vi "PathPlanner_Path_FlipPath.vi"(11 "in PathPlannerPath":T1={"Reversed"=FALSE, "RotationTargets"=[], "ConstraintZones"=[], "EventMarkers"=[], "GlobalConstraints"={"MaxVelocityMps;"=0.0, "MaxAccelerationMpsSq;"=0.0, "MaxAngularVelRadPsEc;"=0.0, "MaxAngularAccRadPSecSq"=0.0, "Exists"=FALSE, "Unlimited"=FALSE, "NominalVoltageVolts"=12.0}, "GoalEndState"={"VelocityMPS"=0.0, "Rotation"={"VALUE"=0.0, "COS"=1.0, "SIN"=0.0}}, "AllPoints"=[], "Name"="", "Waypoints"=[], "PointTowardsZones"=[], "IdealStartingState"={"VelocityMPS"=0.0, "Rotation"={"VALUE"=1.0, "COS"=0.0, "SIN"=0.0}, "NotNull"=FALSE}, "IsChoreoPath"=FALSE, "PreventFlipping"=FALSE} {"IdealStartingState"."Rotation"."SIN" format="%13.4f"; "IdealStartingState"."Rotation"."COS" format="%13.4f"; "IdealStartingState"."Rotation"."VALUE" format="%13.4f"; "PointTowardsZones"."TargetPosition"."Y" format="%14.3f"; "PointTowardsZones"."TargetPosition"."X" format="%14.3f"; "PointTowardsZones"."RotationOffset"."SIN" format="%13.4f"; "PointTowardsZones"."RotationOffset"."COS" format="%13.4f"; "PointTowardsZones"."RotationOffset"."VALUE" format="%13.4f"; "Waypoints"."nextControl"."Y" format="%14.3f"; "Waypoints"."nextControl"."X" format="%14.3f"; "Waypoints"."anchor"."Y" format="%14.3f"; "Waypoints"."anchor"."X" format="%14.3f"; "Waypoints"."prevControl"."Y" format="%14.3f"; "Waypoints"."prevControl"."X" format="%14.3f"; "AllPoints"."RotationTarget"."rotation"."SIN" format="%13.4f"; "AllPoints"."RotationTarget"."rotation"."COS" format="%13.4f"; "AllPoints"."RotationTarget"."rotation"."VALUE" format="%13.4f"; "AllPoints"."Position"."Y" format="%14.3f"; "AllPoints"."Position"."X" format="%14.3f"; "GoalEndState"."Rotation"."SIN" format="%13.4f"; "GoalEndState"."Rotation"."COS" format="%13.4f"; "GoalEndState"."Rotation"."VALUE" format="%13.4f"; "RotationTargets"."rotation"."SIN" format="%13.4f"; "RotationTargets"."rotation"."COS" format="%13.4f"; "RotationTargets"."rotation"."VALUE" format="%13.4f"}) -> (3 "out PathPlannerPath":T1={"Reversed"=FALSE, "RotationTargets"=[], "ConstraintZones"=[], "EventMarkers"=[], "GlobalConstraints"={"MaxVelocityMps;"=0.0, "MaxAccelerationMpsSq;"=0.0, "MaxAngularVelRadPsEc;"=0.0, "MaxAngularAccRadPSecSq"=0.0, "Exists"=FALSE, "Unlimited"=FALSE, "NominalVoltageVolts"=12.0}, "GoalEndState"={"VelocityMPS"=0.0, "Rotation"={"VALUE"=0.0, "COS"=1.0, "SIN"=0.0}}, "AllPoints"=[], "Name"="", "Waypoints"=[], "PointTowardsZones"=[], "IdealStartingState"={"VelocityMPS"=0.0, "Rotation"={"VALUE"=1.0, "COS"=0.0, "SIN"=0.0}, "NotNull"=FALSE}, "IsChoreoPath"=FALSE, "PreventFlipping"=FALSE} {"IdealStartingState"."Rotation"."SIN" format="%13.4f"; "IdealStartingState"."Rotation"."COS" format="%13.4f"; "IdealStartingState"."Rotation"."VALUE" format="%13.4f"; "PointTowardsZones"."TargetPosition"."Y" format="%14.3f"; "PointTowardsZones"."TargetPosition"."X" format="%14.3f"; "PointTowardsZones"."RotationOffset"."SIN" format="%13.4f"; "PointTowardsZones"."RotationOffset"."COS" format="%13.4f"; "PointTowardsZones"."RotationOffset"."VALUE" format="%13.4f"; "Waypoints"."nextControl"."Y" format="%14.3f"; "Waypoints"."nextControl"."X" format="%14.3f"; "Waypoints"."anchor"."Y" format="%14.3f"; "Waypoints"."anchor"."X" format="%14.3f"; "Waypoints"."prevControl"."Y" format="%14.3f"; "Waypoints"."prevControl"."X" format="%14.3f"; "AllPoints"."RotationTarget"."rotation"."SIN" format="%13.4f"; "AllPoints"."RotationTarget"."rotation"."COS" format="%13.4f"; "AllPoints"."RotationTarget"."rotation"."VALUE" format="%13.4f"; "AllPoints"."Position"."Y" format="%14.3f"; "AllPoints"."Position"."X" format="%14.3f"; "GoalEndState"."Rotation"."SIN" format="%13.4f"; "GoalEndState"."Rotation"."COS" format="%13.4f"; "GoalEndState"."Rotation"."VALUE" format="%13.4f"; "RotationTargets"."rotation"."SIN" format="%13.4f"; "RotationTargets"."rotation"."COS" format="%13.4f"; "RotationTargets"."rotation"."VALUE" format="%13.4f"})   [LabVIEW 2019, in "PathPlanner24.lvlib"]
doc: "Flip a path to the other side of the field, maintaining a global blue alliance origin\n\nInputs: \n - Path - cluster - path definition data structure\n\nOutputs:\n - Path - cluster - flipped path"
uses:
  PathPlanner24.lvlib
  TypeDef/PathPlannerPath.ctl
  TypeDef/PathPlannerRotationTarget.ctl
  <vilib>/Rock Robotics/WPI/ThirdParty/JAS_Junk/TrajLib/TypeDef/ROTATION2D.ctl
  TypeDef/PathPlannerConstraintsZone.ctl
  TypeDef/PathPlannerPathConstraints.ctl
  TypeDef/PathPlannerEventMarker.ctl
  TypeDef/PathPlannerCommandUtil.ctl
  ENum/PathPlanner_CommandUtil_Type_ENUM.ctl
  TypeDef/PathPlannerGoalEndState.ctl
  TypeDef/PathPlannerPathPoint.ctl
  <vilib>/Rock Robotics/WPI/ThirdParty/JAS_Junk/TrajLib/TypeDef/TRANSLATION2D.ctl
  TypeDef/PathPlannerWaypoint.ctl
  TypeDef/PathPlannerPointTowardsZone.ctl
  TypeDef/PathPlannerIdealStartingState.ctl
  PathPlanner_FieldUtil_FlipFieldPosition.vi
  PathPlanner_RotationTarget_New.vi
  PathPlanner_RotationTarget_GetAll.vi
  PathPlanner_FieldUtil_FlipFieldRotation.vi
  PathPlanner_FieldUtil_SymmetryType.vi
  PathPlanner_FieldUtil_FieldSizeY.vi
  <vilib>/Rock Robotics/WPI/ThirdParty/JAS_Junk/TrajLib/Translation2d_GetXY.vi
  <vilib>/Rock Robotics/WPI/ThirdParty/JAS_Junk/TrajLib/Translation2d_Create.vi
  PathPlanner_FieldUtil_FieldSizeX.vi
  <vilib>/Rock Robotics/WPI/ThirdParty/JAS_Junk/TrajLib/Rotation2d_CreateAngle.vi
  <vilib>/Rock Robotics/WPI/ThirdParty/JAS_Junk/TrajLib/Rotation2d_Minus.vi
  <vilib>/Rock Robotics/WPI/ThirdParty/JAS_Junk/TrajLib/Conv_Feet_Meters.vi
  <vilib>/Rock Robotics/WPI/ThirdParty/JAS_Junk/TrajLib/Rotation2d_UnaryMinus.vi
  <vilib>/Rock Robotics/WPI/ThirdParty/JAS_Junk/TrajLib/Rotation2d_RotateBy.vi
  <vilib>/Rock Robotics/WPI/ThirdParty/JAS_Junk/TrajLib/Rotation2d_CreateXY.vi
  <vilib>/Rock Robotics/WPI/ThirdParty/JAS_Junk/TrajLib/Util_CalcDist.vi
  <vilib>/Rock Robotics/WPI/ThirdParty/JAS_Junk/TrajLib/Trajectory_Library.lvlib
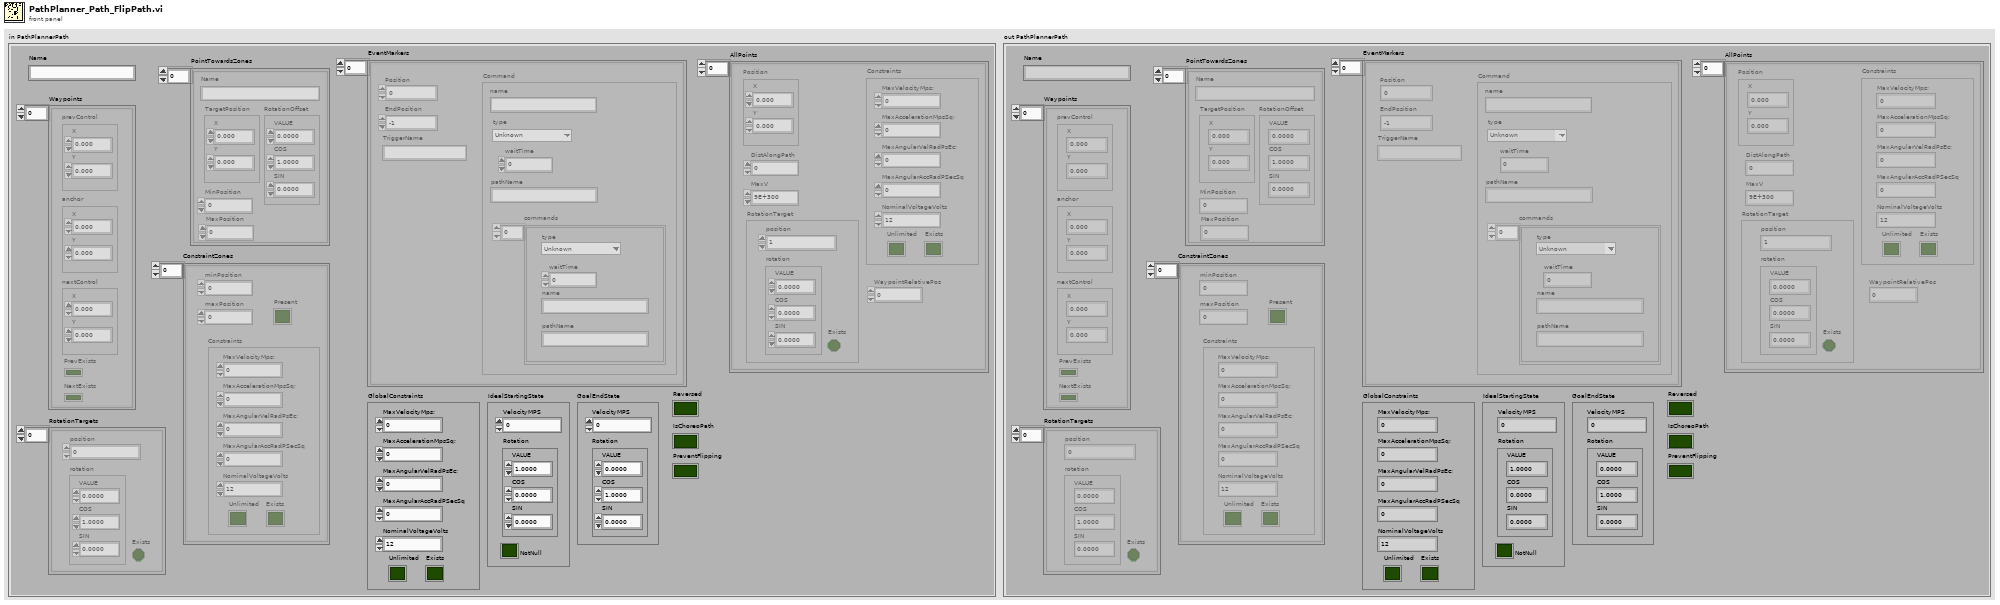
[diagram p1: front panel]
types:
  T1 = typedef "PathPlanner24.lvlib/PathPlannerPath.ctl" = cluster{"Reversed":bool, "RotationTargets":T2[], "ConstraintZones":T4[], "EventMarkers":T6[], "GlobalConstraints":T5, "GoalEndState":T9, "AllPoints":T10[], "Name":string, "Waypoints":T12[], "PointTowardsZones":T13[], "IdealStartingState":T14, "IsChoreoPath":bool, "PreventFlipping":bool}
  T2 = typedef "PathPlanner24.lvlib/PathPlannerRotationTarget.ctl" = cluster{"position":dbl, "rotation":T3, "Exists":bool}
  T3 = typedef "Trajectory_Library.lvlib/ROTATION2D.ctl" = cluster{"VALUE":dbl, "COS":dbl, "SIN":dbl}
  T4 = typedef "PathPlanner24.lvlib/PathPlannerConstraintsZone.ctl" = cluster{"minPosition":dbl, "maxPosition":dbl, "Constraints":T5, "Present":bool}
  T5 = typedef "PathPlanner24.lvlib/PathPlannerPathConstraints.ctl" = cluster{"MaxVelocityMps;":dbl, "MaxAccelerationMpsSq;":dbl, "MaxAngularVelRadPsEc;":dbl, "MaxAngularAccRadPSecSq":dbl, "Exists":bool, "Unlimited":bool, "NominalVoltageVolts":dbl}
  T6 = typedef "PathPlanner24.lvlib/PathPlannerEventMarker.ctl" = cluster{"Position":dbl, "Command":T7, "TriggerName":string, "EndPosition":dbl}
  T7 = typedef "PathPlanner24.lvlib/PathPlannerCommandUtil.ctl" = cluster{"waitTime":dbl, "name":string, "pathName":string, "commands":cluster{"type":T8, "waitTime":dbl, "name":string, "pathName":string}[], "type":T8}
  T8 = typedef "PathPlanner24.lvlib/PathPlanner_CommandUtil_Type_ENUM.ctl" = enum16{"Unknown", "Wait", "Named", "Path", "Sequential", "Parallel", "Race", "Deadline", "PointTowardsZoneEnter", "PointTowardsZoneExit", "TriggerEventStart", "TriggerEventStop", "TriggerEventOneshot"}
  T9 = typedef "PathPlanner24.lvlib/PathPlannerGoalEndState.ctl" = cluster{"VelocityMPS":dbl, "Rotation":T3}
  T10 = typedef "PathPlanner24.lvlib/PathPlannerPathPoint.ctl" = cluster{"Position":T11, "DistAlongPath":dbl, "MaxV":dbl, "Constraints":T5, "RotationTarget":T2, "WaypointRelativePos":dbl}
  T11 = typedef "Trajectory_Library.lvlib/TRANSLATION2D.ctl" = cluster{"X":dbl, "Y":dbl}
  T12 = typedef "PathPlanner24.lvlib/PathPlannerWaypoint.ctl" = cluster{"prevControl":T11, "anchor":T11, "nextControl":T11, "PrevExists":bool, "NextExists":bool}
  T13 = typedef "PathPlanner24.lvlib/PathPlannerPointTowardsZone.ctl" = cluster{"RotationOffset":T3, "Name":string, "TargetPosition":T11, "MinPosition":dbl, "MaxPosition":dbl}
  T14 = typedef "PathPlanner24.lvlib/PathPlannerIdealStartingState.ctl" = cluster{"VelocityMPS":dbl, "Rotation":T3, "NotNull":bool}
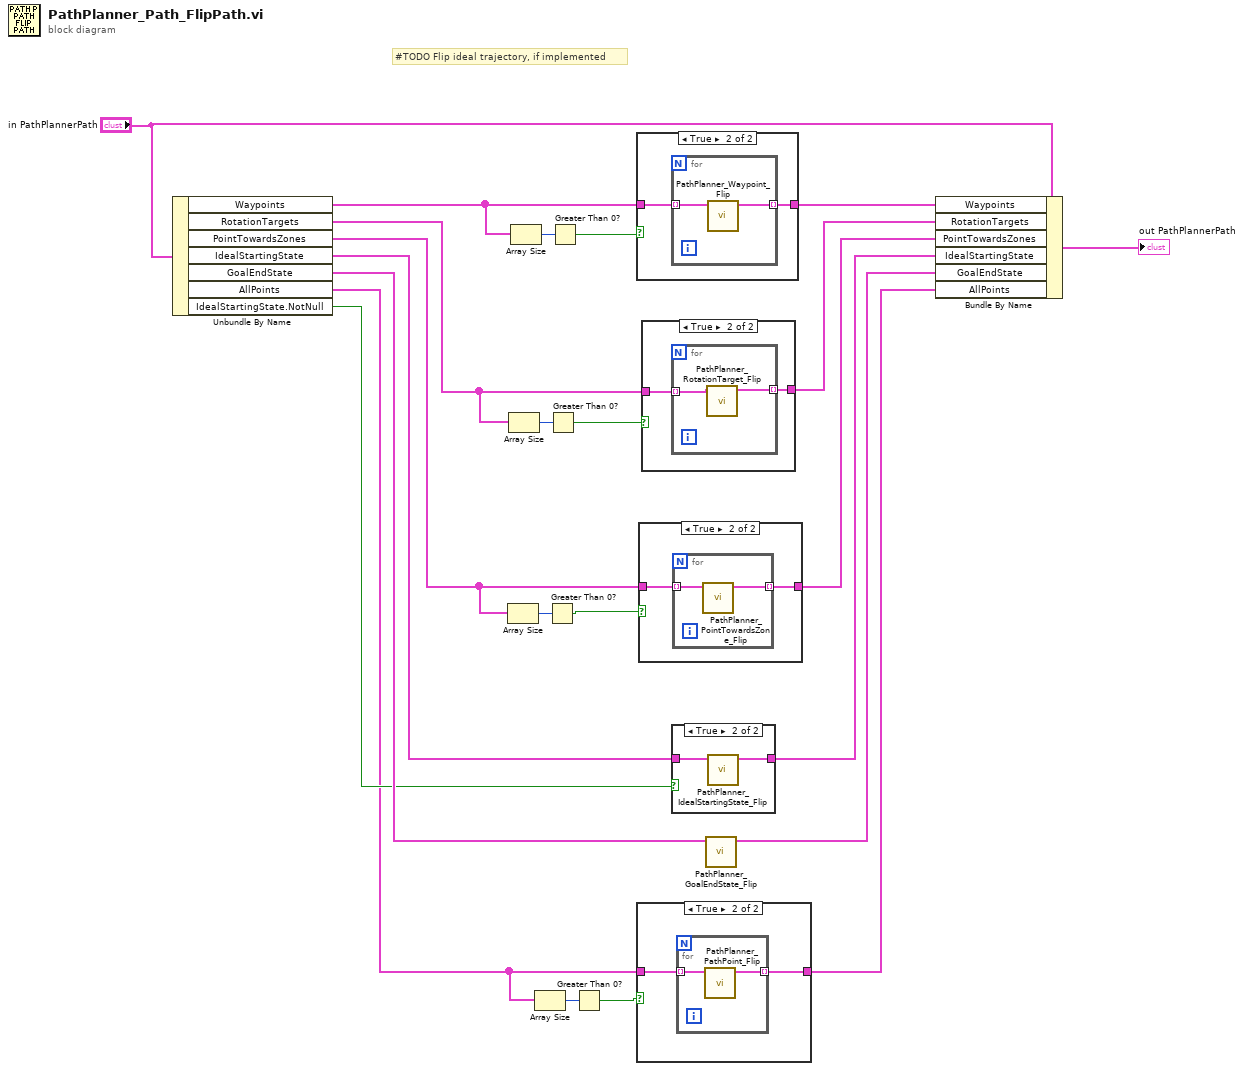
[diagram p0: block diagram]
diagram:
  # "#TODO Flip ideal trajectory, if implemented"
  n1 = Unbundle By Name("in PathPlannerPath") -> ("Waypoints"=w12:T12[], "RotationTargets"=w1:T2[], "PointTowardsZones"=w4:T13[], "IdealStartingState"=w18:T14, "GoalEndState"=w16:T9, "AllPoints"=w6:T10[], "IdealStartingState.NotNull"=w13:bool)
  n2 = Array Size(array=w4) -> (size(s)=w9:i32)
  n3 = Array Size(array=w1) -> (size(s)=w10:i32)
  n4 = Array Size(array=w12) -> (size(s)=w11:i32)
  n5 = Array Size(array=w6) -> (size(s)=w8:i32)
  n6 = Greater Than 0?(x=w9) -> (x > 0?=w5:bool)
  n7 = Greater Than 0?(x=w10) -> (x > 0?=w3:bool)
  n8 = Greater Than 0?(x=w11) -> (x > 0?=w2:bool)
  n9 = Greater Than 0?(x=w8) -> (x > 0?=w7:bool)
  n10 = case shown="True" w2 {
    tunnel: [w24 w26] -> w21
    tunnel: w12 -> [w24 w25]
    frame False {
    }
    frame True {
      n11 = for {
        tunnel: w25 -> [w28] mode=indexing
        tunnel: [w27] -> w26 mode=indexing
        n12 = call "PathPlanner_Waypoint_Flip.vi"("Waypoint"=w28) -> ("FlippedWaypoint"=w27:T12)  [unwired: 10 in]
      }
    }
  }
  n13 = case shown="True" w7 {
    tunnel: w6 -> [w29 w31]
    tunnel: [w29 w30] -> w14
    frame False {
    }
    frame True {
      n14 = for {
        tunnel: w31 -> [w33] mode=indexing
        tunnel: [w32] -> w30 mode=indexing
        n15 = call "PathPlanner_PathPoint_Flip.vi"("PathPlannerPoint"=w33) -> ("FlippedPathPlannerPoint"=w32:T10)  [unwired: 10 in]
      }
    }
  }
  n16 = case shown="True" w5 {
    tunnel: w4 -> [w34 w36]
    tunnel: [w34 w35] -> w19
    frame False {
    }
    frame True {
      n17 = for {
        tunnel: w36 -> [w38] mode=indexing
        tunnel: [w37] -> w35 mode=indexing
        n18 = call "PathPlanner_PointTowardsZone_Flip.vi"("PointTowardsZone"=w38) -> ("FlippedPointTowardsZone"=w37:T13)  [unwired: 10 in]
      }
    }
  }
  n19 = case shown="True" w3 {
    tunnel: w1 -> [w39 w41]
    tunnel: [w39 w40] -> w20
    frame False {
    }
    frame True {
      n20 = for {
        tunnel: w41 -> [w43] mode=indexing
        tunnel: [w42] -> w40 mode=indexing
        n21 = call "PathPlanner_RotationTarget_Flip.vi"("RotationTarget"=w43) -> ("FlippedRotationTarget"=w42:T2)  [unwired: 10 in]
      }
    }
  }
  n22 = case shown="True" w13 {
    tunnel: w18 -> [w44 w46]
    tunnel: [w44 w45] -> w17
    frame False {
    }
    frame True {
      n23 = call "PathPlanner_IdealStartingState_Flip.vi"("IdealStartingState"=w46) -> ("FlippedIdealStartingState"=w45:T14)  [unwired: 10 in]
    }
  }
  n24 = call "PathPlanner_GoalEndState_Flip.vi"("GoalEndState"=w16) -> ("FlippedGoalEndState"=w15:T9)  [unwired: 10 in]
  n25 = Bundle By Name(cluster="in PathPlannerPath", "Waypoints"=w21, "RotationTargets"=w20, "PointTowardsZones"=w19, "IdealStartingState"=w17, "GoalEndState"=w15, "AllPoints"=w14) -> (→"out PathPlannerPath":T1)
